vi "ScaleAI16_gen.vi"(0 "M":sgl[](array[numeric])=[0.0, 0.0, 0.0, 0.0, 0.0, 0.0, 0.0, 0.0, 0.0, 0.0, 0.0, 0.0, 0.0, 0.0, 0.0, 0.0], 5 "B":i16[](array[numeric])=[0, 0, 0, 0, 0, 0, 0, 0, 0, 0, 0, 0, 0, 0, 0, 0], 7 "UnscaledAI":i16[](array[numeric])=[0, 0, 0, 0, 0, 0, 0, 0, 0, 0, 0, 0, 0, 0, 0, 0], 9 "input valid":bool=TRUE) -> (4 "ScaledAI":sgl[](array[numeric]), 10 "output valid":bool, 14 "feedback signals":cluster{"ready for input":bool})   [LabVIEW 2015]
doc: "This VI is created by the NI LabVIEW 2015 FPGA IP Builder.\n\nProject: ScaleAndLimit.lvproj\nTarget: FPGA Target (sbRIO-9607)/IP Builder\nBuild Specification: ScaleAI16_src\nDirectives Item: ScaleAI16_src\nTop-Level VI: C:\\LabVIEWPowerElectronicsControl\\ScaleAndLimit\\dev\\Core\\IPBuilder\\ScaleAI16_src.vi\n\nQuick Device Utilization Estimate\n--------------------------------------------\nSlice Registers: 2.3% (2425 out of 106400)\nSlice LUTs: 10.0% (5337 out of 53200)\nDSP48s: 1.4% (3 out of 220)\nBlock RAMs: 0.0% (0 out of 280)\n\nQuick Performance Estimate\n--------------------------------------------\nClock rate (MHz): 47.71\nInitiation interval (cycles): 36\nPipeline type: Not pipelined\nMinimum latency: 35\nMaximum latency: 35"
uses:
  <vilib>/rvi/IPIntegrationNode/IPINode_Typedef/niFpgaIPINodeSupportedFamilies.ctl
  <vilib>/rvi/IPIntegrationNode/IPINode_Utilities/niFpgaIPINodeSimCore.vi
  <vilib>/rvi/IPIntegrationNode/IPINode_Xnode/niFpgaIPINode.xnode
  <vilib>/NI/PowerElectronicsControl/ScaleAndLimit/Core/IPBuilder/ScaleAI16_gen Support/IPBlockSimFiles/xsim.dir/mFE612D4E_topH/xsimkB83B4C7EC23A41F6932D71BE84E7BAB7.dll
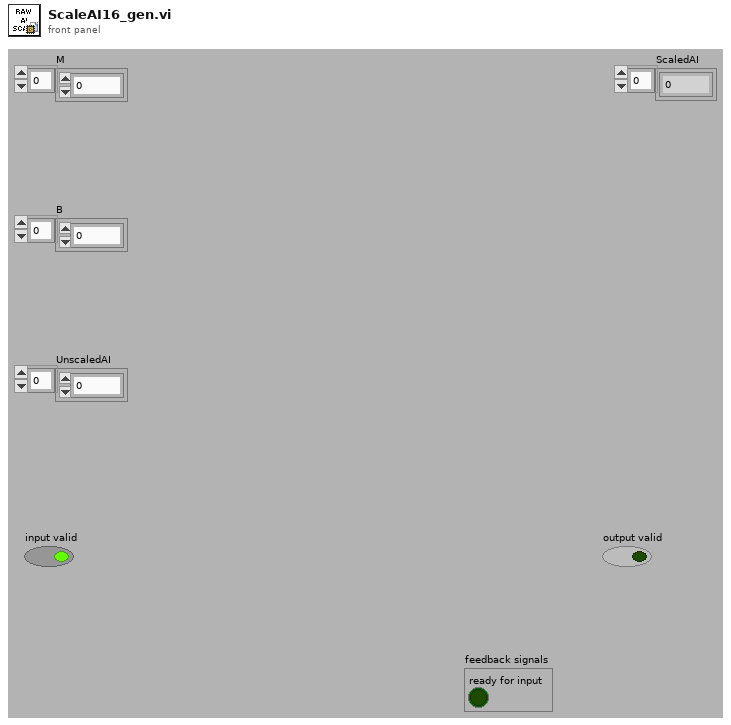
[diagram p1: front panel]
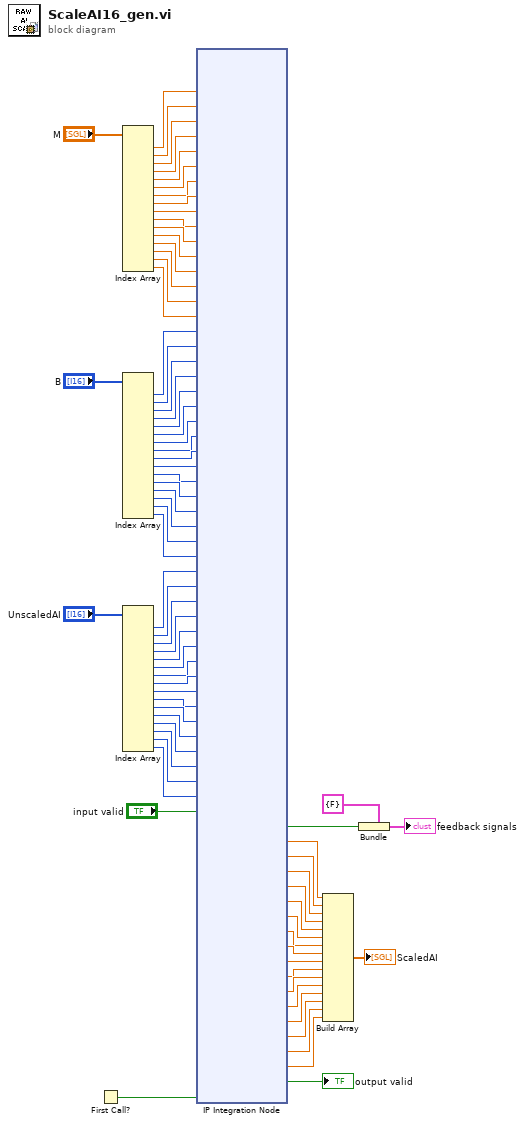
[diagram p0: block diagram]
diagram:
  n1 = First Call?() -> (First Call?: T/F=w74:bool)
  n2 = Index Array(array="M") -> (element #1=w49:sgl, element #2=w50:sgl, element #3=w51:sgl, element #4=w52:sgl, element #5=w53:sgl, element #6=w54:sgl, element #7=w55:sgl, element #8=w56:sgl, element #9=w57:sgl, element #10=w58:sgl, element #11=w59:sgl, element #12=w60:sgl, element #13=w61:sgl, element #14=w62:sgl, element #15=w63:sgl, element #16=w64:sgl)  [unwired: 16 in]
  n3 = Index Array(array="B") -> (element #1=w33:i16, element #2=w34:i16, element #3=w35:i16, element #4=w36:i16, element #5=w37:i16, element #6=w38:i16, element #7=w39:i16, element #8=w40:i16, element #9=w41:i16, element #10=w42:i16, element #11=w43:i16, element #12=w44:i16, element #13=w45:i16, element #14=w46:i16, element #15=w47:i16, element #16=w48:i16)  [unwired: 16 in]
  n4 = Index Array(array="UnscaledAI") -> (element #1=w17:i16, element #2=w18:i16, element #3=w19:i16, element #4=w20:i16, element #5=w21:i16, element #6=w22:i16, element #7=w23:i16, element #8=w24:i16, element #9=w25:i16, element #10=w26:i16, element #11=w27:i16, element #12=w28:i16, element #13=w29:i16, element #14=w30:i16, element #15=w31:i16, element #16=w32:i16)  [unwired: 16 in]
  n5 = xnode "IP Integration Node"("p_9_M_0"=w49, "p_9_M_1"=w50, "p_9_M_2"=w51, "p_9_M_3"=w52, "p_9_M_4"=w53, "p_9_M_5"=w54, "p_9_M_6"=w55, "p_9_M_7"=w56, "p_9_M_8"=w57, "p_9_M_9"=w58, "p_9_M_10"=w59, "p_9_M_11"=w60, "p_9_M_12"=w61, "p_9_M_13"=w62, "p_9_M_14"=w63, "p_9_M_15"=w64, "p_7_B_0"=w33, "p_7_B_1"=w34, "p_7_B_2"=w35, "p_7_B_3"=w36, "p_7_B_4"=w37, "p_7_B_5"=w38, "p_7_B_6"=w39, "p_7_B_7"=w40, "p_7_B_8"=w41, "p_7_B_9"=w42, "p_7_B_10"=w43, "p_7_B_11"=w44, "p_7_B_12"=w45, "p_7_B_13"=w46, "p_7_B_14"=w47, "p_7_B_15"=w48, "p_0_UnscaledAI_0"=w17, "p_0_UnscaledAI_1"=w18, "p_0_UnscaledAI_2"=w19, "p_0_UnscaledAI_3"=w20, "p_0_UnscaledAI_4"=w21, "p_0_UnscaledAI_5"=w22, "p_0_UnscaledAI_6"=w23, "p_0_UnscaledAI_7"=w24, "p_0_UnscaledAI_8"=w25, "p_0_UnscaledAI_9"=w26, "p_0_UnscaledAI_10"=w27, "p_0_UnscaledAI_11"=w28, "p_0_UnscaledAI_12"=w29, "p_0_UnscaledAI_13"=w30, "p_0_UnscaledAI_14"=w31, "p_0_UnscaledAI_15"=w32, "input_valid"="input valid", "first_call"=w74) -> ("ready_for_input"=w71:bool, "p_4_ScaledAI_0"=w1:sgl, "p_4_ScaledAI_1"=w2:sgl, "p_4_ScaledAI_2"=w3:sgl, "p_4_ScaledAI_3"=w4:sgl, "p_4_ScaledAI_4"=w5:sgl, "p_4_ScaledAI_5"=w6:sgl, "p_4_ScaledAI_6"=w7:sgl, "p_4_ScaledAI_7"=w8:sgl, "p_4_ScaledAI_8"=w9:sgl, "p_4_ScaledAI_9"=w10:sgl, "p_4_ScaledAI_10"=w11:sgl, "p_4_ScaledAI_11"=w12:sgl, "p_4_ScaledAI_12"=w13:sgl, "p_4_ScaledAI_13"=w14:sgl, "p_4_ScaledAI_14"=w15:sgl, "p_4_ScaledAI_15"=w16:sgl, "output_valid"=→"output valid":bool)  [unwired: 2 in]
  n6 = Build Array(w1, w2, w3, w4, w5, w6, w7, w8, w9, w10, w11, w12, w13, w14, w15, w16) -> (→"ScaledAI":sgl[])
  n7 = Bundle ("Bundle_feedback")(cluster=cluster{"ready for input":bool} {"ready for input"=FALSE}, "ready for input"=w71) -> (→"feedback signals":cluster{"ready for input":bool})
